vi "DrawTiles.vi"() -> ()   [LabVIEW 2019, in "Initializers.lvlib"]
uses:
  Initializers.lvlib
  <vilib>/Utility/miscctls.llb/LVPoint32TypeDef.ctl
  <vilib>/Utility/miscctls.llb/LVBoundsTypeDef.ctl
  <vilib>/picture/picture.llb/imagedata.ctl
panel:
  out "new picture 3":picture
  out "TileIndex":u8
  in  "TileNo_y":u8
  out "new picture 2":picture
  in  "TileNo_x":u8
  in  "path to PNG file":path
  in  "stop":bool
  out "Coords":T1
  out "new picture":picture
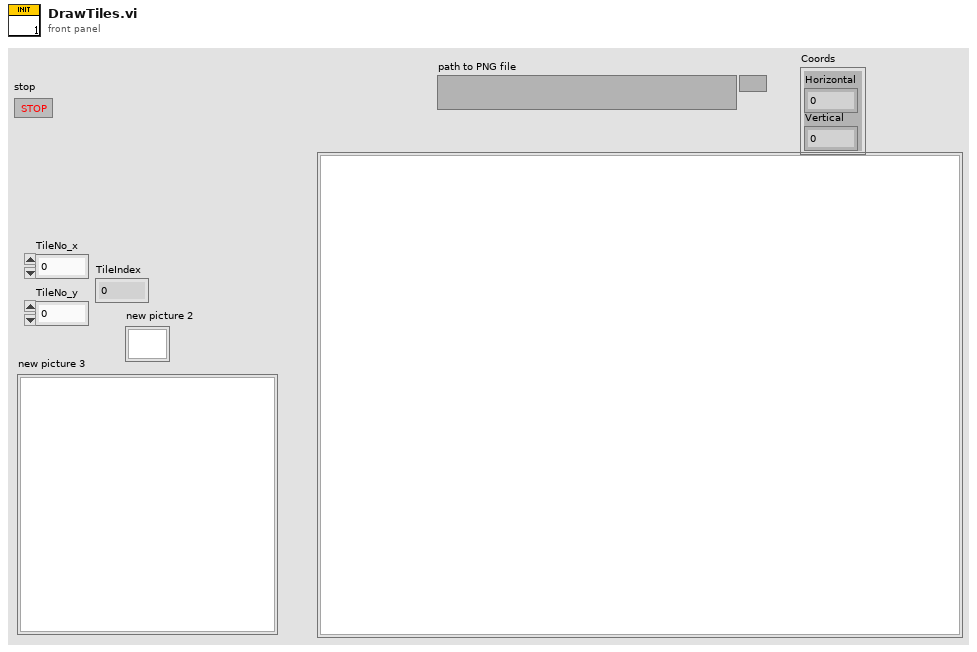
[diagram p1: front panel]
types:
  T1 = typedef "LVPoint32TypeDef.ctl" = cluster{"Horizontal":i32, "Vertical":i32}
  T2 = typedef "imagedata.ctl" = cluster{"image type":i32, "image depth":i32, "image":u8[], "mask":u8[], "colors":u32[], "Rectangle":cluster{"left":i16, "top":i16, "right":i16, "bottom":i16}}
  T3 = typedef "LVBoundsTypeDef.ctl" = cluster{"Width":u32, "Height":u32}
  T4 = cluster{"left":i16, "top":i16, "right":i16, "bottom":i16}
  T5 = typedef "LVPositionTypeDef.ctl" = cluster{"Left":i32, "Top":i32}
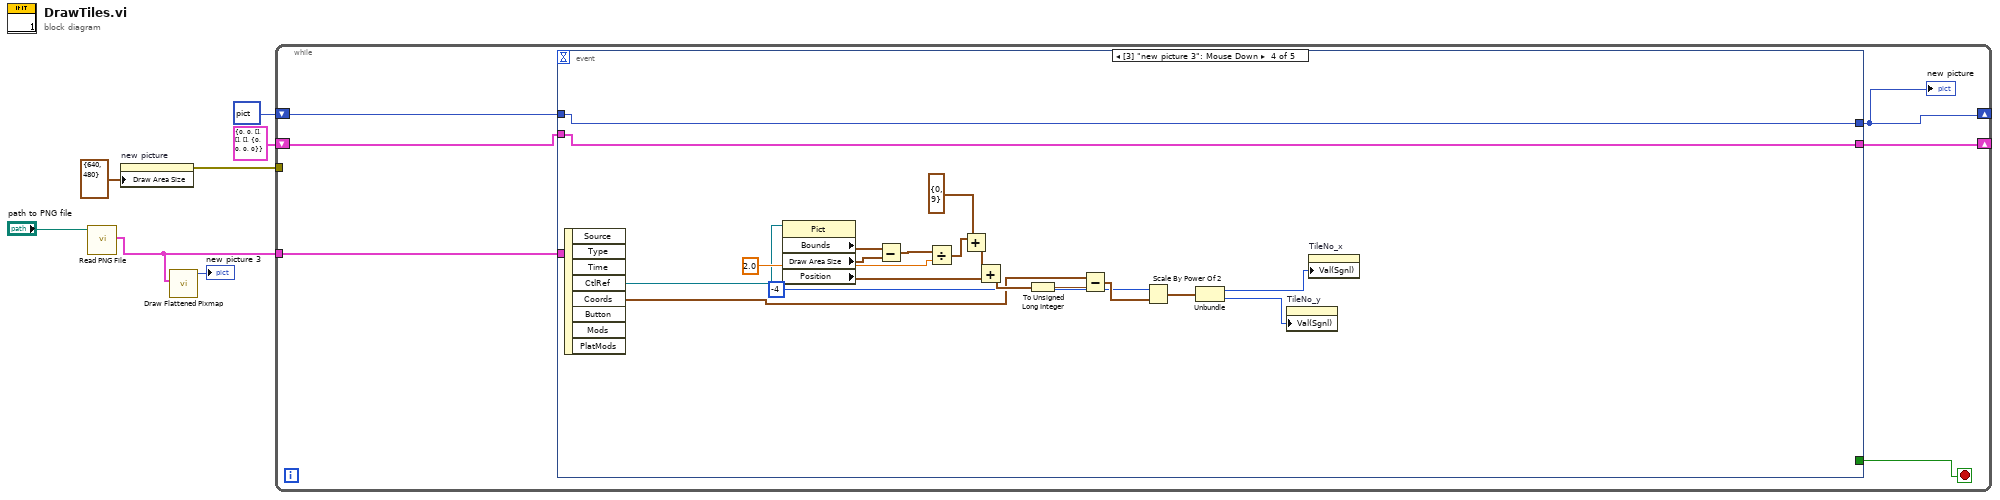
[diagram p0: block diagram]
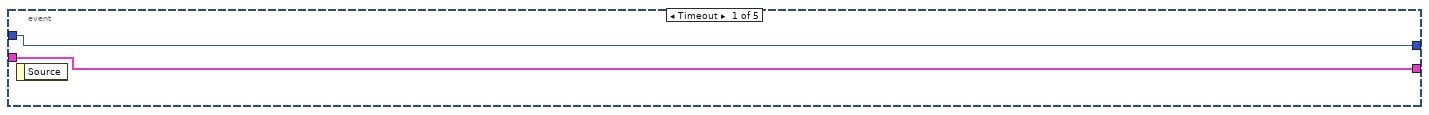
[diagram p2: hidden frame]
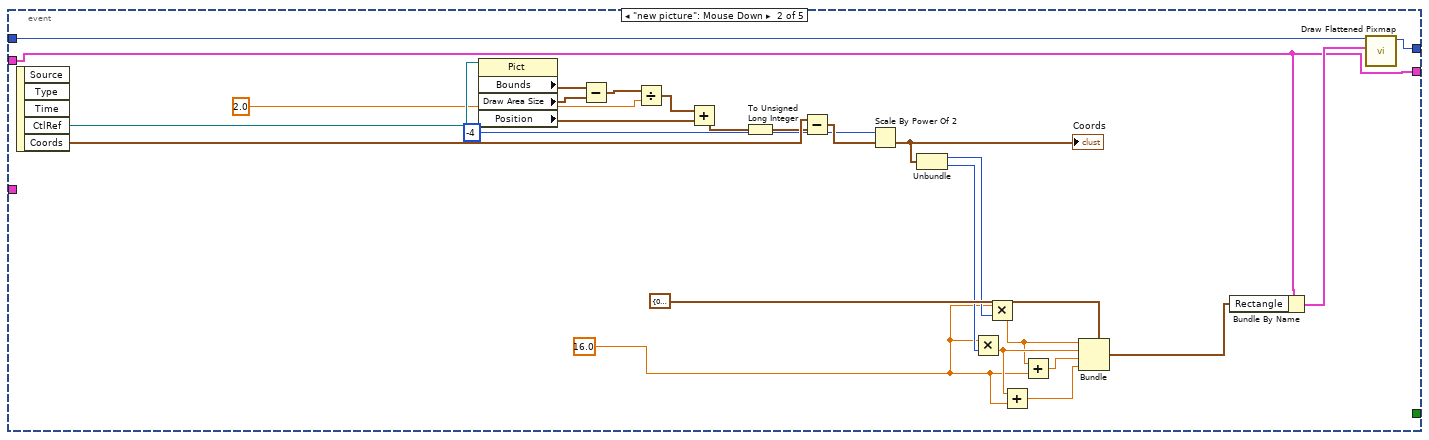
[diagram p3: hidden frame]
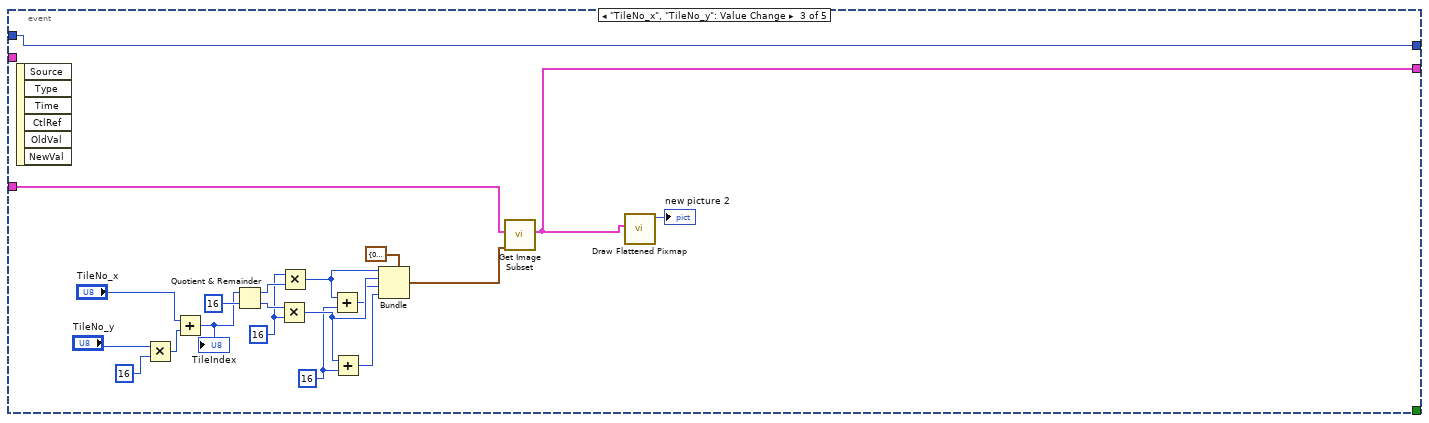
[diagram p4: hidden frame]
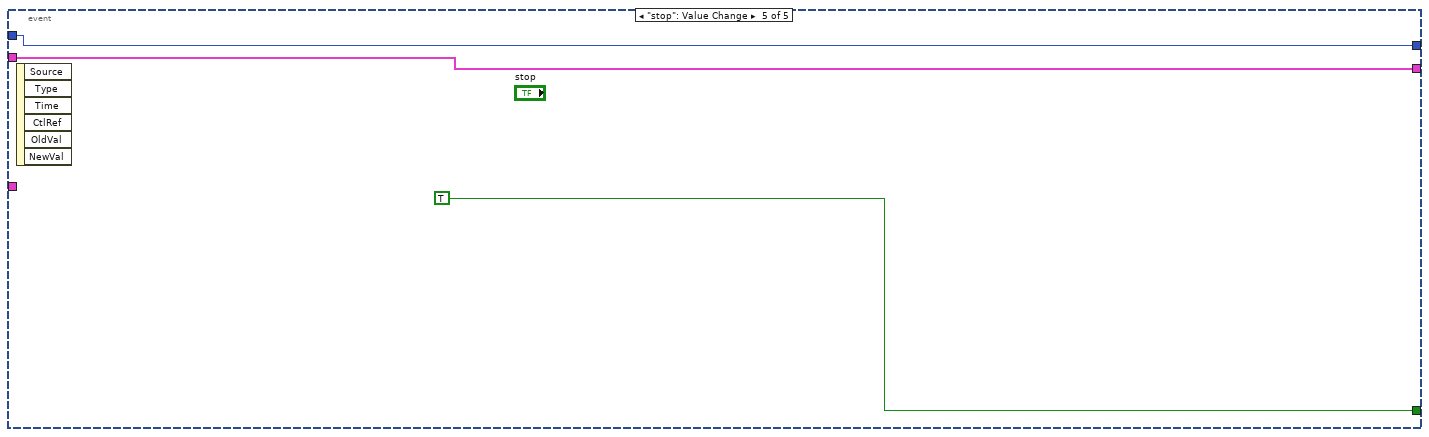
[diagram p5: hidden frame]
diagram:
  n1 = call <vilib>:"Read PNG File.vi"("path to PNG file"="path to PNG file") -> ("image data"=w2:T2)  [unwired: 8 in, 2 out]
  n2 = property on="new picture" class="Pict"("Draw Area Size"=T3 {"Width"=640, "Height"=480}) -> (error out=w6:errorcluster)  [unwired: 2 in, 1 out]
  n3 = call <vilib>:"Draw Flattened Pixmap.vi"("image data"=w2) -> ("new picture"=→"new picture 3":picture)  [unwired: 8 in]
  n4 = while {
    tunnel: w6 -> [_]
    shift-right: [w10] -> _
    shift-left: picture bytes[189126] ("new picture") -> [w12]
    tunnel: w2 -> [w11]
    shift-right: [w9] -> _
    shift-left: T2 {"image type"=0, "image depth"=0, "image"=[], "mask"=[], "colors"=[], "Rectangle"={"left"=0, "top"=0, "right"=0, "bottom"=0}} ("image subset") -> [w8]
    stop <- w13 stop-if-true
    n5 = event shown="[3] \"new picture 3\": Mouse Down" {
      selector: _ -> [_ _ _ _ _]
      dyn-events: _ -> [_ _ _ _ _]
      timeout: _ -> [_ _ _ _ _]
      tunnel: [_ _ _ _ TRUE] -> w13
      tunnel: w12 -> [w15 w28 w60 w80 w82]
      tunnel: w11 -> [_ _ w61 _ _]
      tunnel: [w15 w27 w60 w80 w82] -> w10
      tunnel: [w14 w16 w49 w79 w81] -> w9
      tunnel: w8 -> [w14 w16 _ w79 w81]
      event Timeout {
        n6 = event-data() -> ()  [unwired: 1 in, 1 out]
      }
      event "new picture": Mouse Down {
        w19 = 16.0 ("y")
        n7 = event-data() -> ("CtlRef"=w41:refnum<vi>, "Coords"=w40:T1)  [unwired: 1 in, 3 out]
        n8 = property class="Pict"(reference=w41) -> ("Bounds"=w36:T3, "Draw Area Size"=w35:T3, "Position"=w37:T5)  [unwired: 1 in, 2 out]
        n9 = Subtract(x=w36, y=w35) -> (x-y=w34:T3)
        n10 = Divide(x=w34, y=2.0) -> (x/y=w32:cluster{"Width":dbl, "Height":dbl})
        n11 = Add(x=w32, y=w37) -> (x+y=w38:cluster{dbl, dbl})
        n12 = To Unsigned Long Integer(number=w38) -> (unsigned 32bit integer=w21:cluster{u32, u32})
        n13 = Subtract(x=w40, y=w21) -> (x-y=w39:cluster{u32, u32})
        n14 = Scale By Power Of 2(n=i16 -4, x=w39) -> (x*2^n=w30:cluster{u32, u32})
        "Coords" <- w30
        n15 = Unbundle(w30) -> (w25:u32, w24:u32)
        n16 = Multiply(x=w19, y=w24) -> (x*y=w22:dbl)
        n17 = Multiply(x=w19, y=w25) -> (x*y=w20:dbl)
        n18 = Add(x=w22, y=w19) -> (x+y=w26:dbl)
        n19 = Add(x=w20, y=w19) -> (x+y=w23:dbl)
        n20 = Bundle(cluster=T4 {"left"=0, "top"=0, "right"=0, "bottom"=0} ("subset rect"), "left"=w20, "top"=w22, "right"=w23, "bottom"=w26) -> (w18:T4)
        n21 = Bundle By Name(cluster=w16, "Rectangle"=w18) -> (w17:T2)
        n22 = call <vilib>:"Draw Flattened Pixmap.vi"("image data"=w17, "picture"=w28) -> ("new picture"=w27:picture)  [unwired: 7 in]
      }
      event "TileNo_x", "TileNo_y": Value Change {
        w53 = u8 16 ("y")
        w52 = u8 16 ("y")
        n23 = event-data() -> ()  [unwired: 1 in, 6 out]
        n24 = Multiply(x="TileNo_y", y=u8 16) -> (x*y=w45:u8)
        n25 = Add(x="TileNo_x", y=w45) -> (x+y=w43:u8)
        "TileIndex" <- w43
        n26 = Quotient & Remainder(x=w43, y=u8 16) -> (x-y*floor(x/y)=w58:u8, floor(x/y)=w59:u8)
        n27 = Multiply(x=w59, y=w52) -> (x*y=w55:u8)
        n28 = Multiply(x=w52, y=w58) -> (x*y=w57:u8)
        n29 = Add(x=w57, y=w53) -> (x+y=w54:u8)
        n30 = Add(x=w55, y=w53) -> (x+y=w56:u8)
        n31 = Bundle(cluster=T4 {"left"=0, "top"=0, "right"=0, "bottom"=0} ("subset rect"), "left"=w57, "top"=w55, "right"=w54, "bottom"=w56) -> (w50:T4)
        n32 = call <vilib>:"Get Image Subset.vi"("subset rect"=w50, "image data"=w61) -> ("image subset"=w49:T2)  [unwired: 4 in, 1 out]
        n33 = call <vilib>:"Draw Flattened Pixmap.vi"("image data"=w49) -> ("new picture"=→"new picture 2":picture)  [unwired: 8 in]
      }
      event "new picture 3": Mouse Down {
        n34 = event-data() -> ("CtlRef"=w68:refnum<vi>, "Coords"=w67:T1)  [unwired: 1 in, 6 out]
        n35 = property class="Pict"(reference=w68) -> ("Bounds"=w75:T3, "Draw Area Size"=w74:T3, "Position"=w76:T5)  [unwired: 1 in, 2 out]
        n36 = Subtract(x=w75, y=w74) -> (x-y=w73:T3)
        n37 = Divide(x=w73, y=2.0) -> (x/y=w71:cluster{"Width":dbl, "Height":dbl})
        n38 = Add(x=w71, y=cluster{"Width":u16, "Height":u16} {"Width"=0, "Height"=9} ("x")) -> (x+y=w63:cluster{"Width":dbl, "Height":dbl})
        n39 = Add(x=w63, y=w76) -> (x+y=w77:cluster{dbl, dbl})
        n40 = To Unsigned Long Integer(number=w77) -> (unsigned 32bit integer=w69:cluster{u32, u32})
        n41 = Subtract(x=w67, y=w69) -> (x-y=w78:cluster{u32, u32})
        n42 = Scale By Power Of 2(n=i16 -4, x=w78) -> (x*2^n=w66:cluster{u32, u32})
        n43 = Unbundle(w66) -> (w65:u32, w64:u32)
        n44 = property on="TileNo_y" class="DigNum (strict)"("Val(Sgnl)"=w64) -> ()  [unwired: 2 in, 2 out]
        n45 = property on="TileNo_x" class="DigNum (strict)"("Val(Sgnl)"=w65) -> ()  [unwired: 2 in, 2 out]
      }
      event "stop": Value Change {
        n46 = event-data() -> ()  [unwired: 1 in, 6 out]
      }
    }
    "new picture" <- w10
  }
